vi "Configure Datalogger.vi"(8 "error in (no error)":errorcluster, 10 "Base File Path":path, 11 "Datalogger Actor in":refnum<class "Datalogger Actor.lvclass">) -> (0 "error out":errorcluster, 3 "Datalogger Actor out":refnum<class "Datalogger Actor.lvclass">)   [LabVIEW 2018, in "Datalogger Actor.lvlib" / "Datalogger Actor.lvclass"]
uses:
  Datalogger Actor.lvclass
  C:/Program Files (x86)/National Instruments/LabVIEW 2018/vi.lib/ActorFramework/Actor/Actor.lvclass
  Datalogger Actor.lvclass/Datalogger Actor.ctl
  <vilib>/ActorFramework/Actor/Actor.lvclass/Actor.ctl
  <vilib>/ActorFramework/Message Enqueuer/Message Enqueuer.lvclass/Message Enqueuer.ctl
  <vilib>/ActorFramework/Message Enqueuer/Init from Existing Queue.vi
  <vilib>/ActorFramework/Message Enqueuer/Message Enqueuer.lvclass
  <vilib>/ActorFramework/Actor/Actor.lvclass
  Datalogger Actor Messages/Open Log File Msg/Open Log File Msg.lvclass
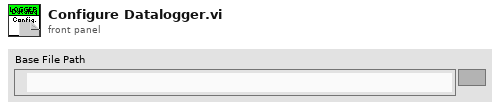
[diagram p1: front panel]
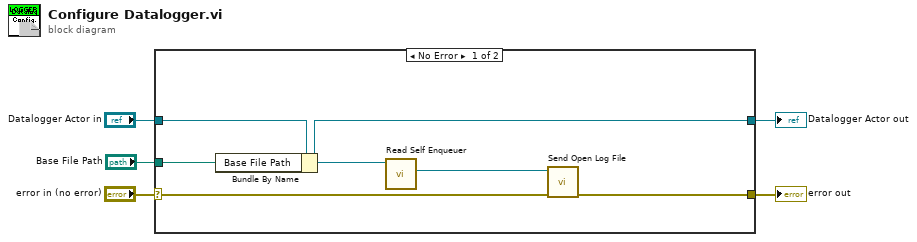
[diagram p0: block diagram]
diagram:
  n1 = case shown="No Error" "error in (no error)" {
    selector: "error in (no error)" -> [w9 w13]
    tunnel: [w8 w13] -> w4
    tunnel: [w6 w12] -> w2
    tunnel: "Datalogger Actor in" -> [w10 w12]
    tunnel: "Base File Path" -> [w11 _]
    frame No Error {
      n2 = Bundle By Name(cluster=w10, "Base File Path"=w11) -> (w6:refnum<class "Datalogger Actor.lvclass">)
      n3 = call <vilib>:"Read Self Enqueuer.vi"("Actor"=w6) -> ("Self Enqueuer"=w7:refnum<class "Message Enqueuer.lvclass">)  [unwired: 10 in]
      n4 = call "Send Open Log File.vi"("error in (no error)"=w9, "Message Enqueuer in"=w7) -> ("error out"=w8:errorcluster)  [unwired: 8 in, 1 out]
    }
    frame Error {
    }
  }
  "error out" <- w4
  "Datalogger Actor out" <- w2
